vi "ConfigMessageMetadata.vi"(9 "TellOrigin":T1, 10 "Lifetime":T3, 11 "ActorAlias":string) -> (3 "MessageMetadata":T2 {"AbsoluteTime" format="%<%x %.3X>T"})   [LabVIEW 2020, in "jettl.lvlib"]
uses:
  jettl.lvlib
  Lifecycle.ctl
  MessageMetadata.ctl
  TellOrigin.ctl
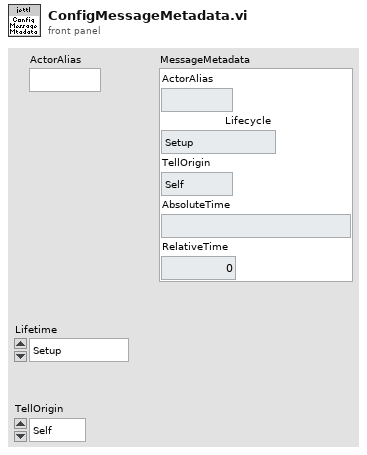
[diagram p1: front panel]
types:
  T1 = typedef "jettl.lvlib/TellOrigin.ctl" = enum16{"Self", "Mediator", "Component"}
  T2 = typedef "jettl.lvlib/MessageMetadata.ctl" = cluster{"ActorAlias":string, "Lifecycle":T3, "TellOrigin":T1, "AbsoluteTime":timestamp, "RelativeTime":dbl}
  T3 = typedef "jettl.lvlib/Lifecycle.ctl" = enum16{"Setup", "TeardownBeforeStart", "Start", "Running", "Stop", "TeardownAfterStart"}
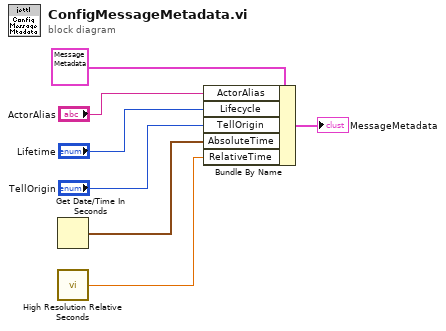
[diagram p0: block diagram]
diagram:
  n1 = Get Date/Time In Seconds() -> (seconds since 1Jan1904=w6:timestamp)
  n2 = call <vilib>:"High Resolution Relative Seconds.vi"() -> ("relative seconds"=w7:dbl)
  n3 = Bundle By Name(cluster=T2 {"ActorAlias"="", "Lifecycle"=enum."Setup", "TellOrigin"=enum."Self", "AbsoluteTime"=timestamp(0 s since 1904-01-01), "RelativeTime"=0.0} ("MessageMetadata"), "ActorAlias"="ActorAlias", "Lifecycle"="Lifetime", "TellOrigin"="TellOrigin", "AbsoluteTime"=w6, "RelativeTime"=w7) -> (→"MessageMetadata":T2)
